vi "System Log Builder (SubVI).vi"(9 "String in":string, 10 "System Uptime":string, 11 "date/time string":string) -> (3 "String out":string)   [LabVIEW 2017]
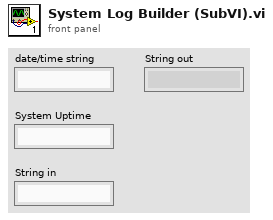
[diagram p1: front panel]
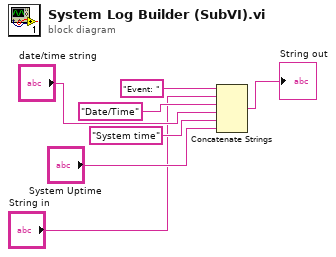
[diagram p0: block diagram]
diagram:
  n1 = Concatenate Strings("Event: ", "String in", "Date/Time", "date/time string", "System time", "System Uptime") -> (→"String out":string)
